vi "PH_USB600x_AnalogReader.set timing mode.vi"(0 "i ref in":refnum<vi>, 1 "Samples per Channel":i32=1000, 2 "Rate":dbl=10000.0 caption="Rate (Hz)" format="%0.2f", 5 "error in (no error)":errorcluster) -> (14 "i ref out":refnum<vi>, 19 "error out":errorcluster)   [LabVIEW 2014, in "PH_USB600x_AnalogReader.lvlib"]
doc: "Sets the timing mode for the scope.\n\nLicense Agreement for this software:\n\nCopyright (C)\nGesellschaft für Schwerionenforschung, GSI\nPlanckstr. 1\n64291 Darmstadt\nGermany\n\nContact: D.Beck@gsi.de \n\nThis program is free software; you can redistribute it and/or modify it under the terms of the GNU General Public License as published by the Free Software Foundation; either version 2 of the license, or (at your option) any later version.\n\nThis program is distributed in the hope that it will be useful, but WITHOUT ANY WARRANTY; without even the implied warranty of MERCHANTABILITY or FITNESS FOR A PARTICULAR PURPOSE. See the GNU General License for more details (http://www.gnu.org).\n\nGesellschaft für Schwerionenforschung, GSI\nPlanckstr. 1, 64291 Darmstadt, Germany\nFor all questions and ideas contact: M.Richter@gsi.de, H.Brand@gsi.de or D.Beck@gsi.de.\nLast update: 17-JUN-2004"
uses:
  PH_USB600x_AnalogReader.lvlib
  PH_Basics/PH_StatusHandler/PH_StatusHandler.Status.ctl
  <vilib>/DAQmx/configure/timing.llb/DAQmx Timing (Sample Clock).vi
  PH_Basics/PH_StatusHandler/PH_StatusHandler.lvlib
  PH_Basics/PH_Common/PH_Common.lvlib
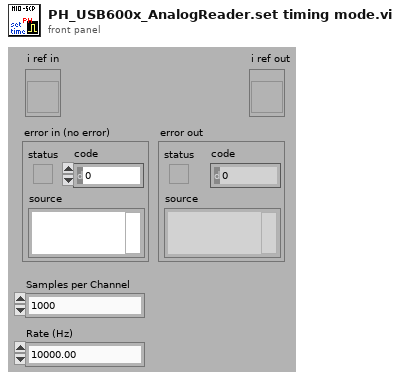
[diagram p1: front panel]
types:
  T1 = typedef "PH_USB600x_AnalogReader.lvlib/PH_USB600x_AnalogReader.i attribute.ctl" = cluster{"GUI Refs":cluster{"Delete":refnum<vi>, "Status":refnum<vi>, "Timeout":refnum<vi>, "Acquire Waveform":refnum<vi>, "Timing":refnum<vi>, "Graph":refnum<vi>, "Prdc Interval":refnum<vi>, "Formula":refnum<vi>}, "Device Settings":cluster{"AIChannel":refnum<k21>, "channelName":string, "Status":T2}, "Timing":T3, "Prdc Interval":dbl, "Lin Scaling":T4, "Data":cluster{"t0":timestamp, dbl}[]}
  T2 = typedef "PH_StatusHandler.lvlib/PH_StatusHandler.Status.ctl" = i16
  T3 = typedef "PH_USB600x_AnalogReader.lvlib/PH_USB600x_AnalogReader.Timing.ctl" = cluster{"Samples per Channel":i32, "Rate":dbl}
  T4 = typedef "PH_USB600x_AnalogReader.lvlib/PH_USB600x_AnalogReader.Lin Scaling.ctl" = cluster{"Slope [Unit/V]":dbl, "Offset [Unit]":dbl, "Y-Unit":string, "Y-Label":string}
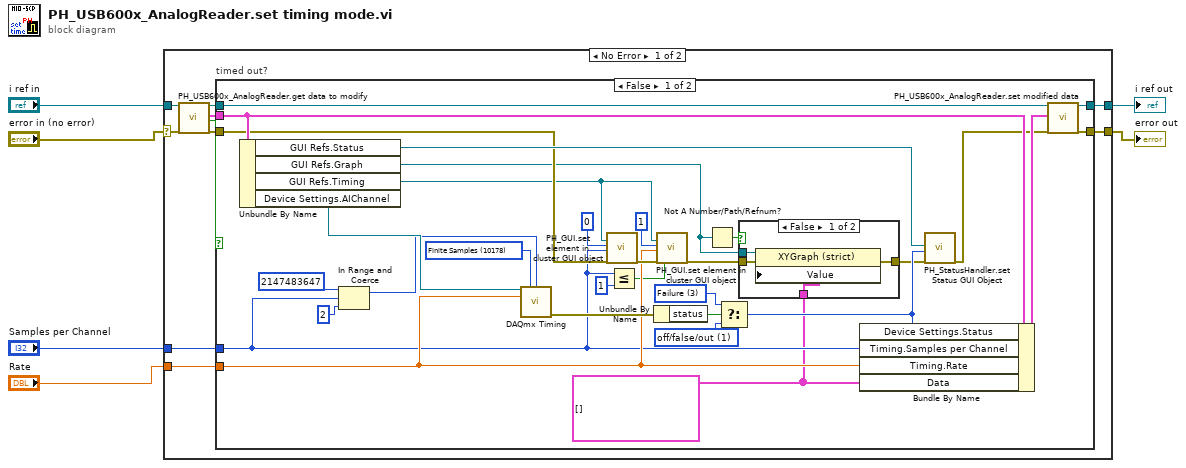
[diagram p0: block diagram]
diagram:
  n1 = case shown="No Error" "error in (no error)" {
    selector: "error in (no error)" -> [w7 w55]
    tunnel: "i ref in" -> [w16 w56]
    tunnel: [w14 w56] -> w5
    tunnel: [w12 w55] -> w4
    tunnel: "Samples per Channel" -> [w9 _]
    tunnel: "Rate" -> [w8 _]
    frame No Error {
      n2 = call "PH_USB600x_AnalogReader.get data to modify.vi"("i ref in"=w16, "error in (no error)"=w7) -> ("i ref out"=w15:refnum<vi>, "i attribute"=w10:T1, "timed out"=w11:bool, "error out"=w13:errorcluster)  [unwired: 14 in]
      n3 = case "timed out?" shown="False" w11 {
        tunnel: [w45 w54] -> w14
        tunnel: w15 -> [w42 w54]
        tunnel: [w41 w53] -> w12
        tunnel: w13 -> [w33 w53]
        tunnel: w10 -> [w44 _]
        tunnel: w9 -> [w23 _]
        tunnel: w8 -> [w31 _]
        frame False {
          w17 = cluster{"t0":timestamp, dbl}[] [] ("Data")
          w38 = T2 1 items=["no info", "off/false/out", "on/true/in", "Failure", "Alarm", "Status 1", "Status 2", "Status 3"] ("Device Settings.Status")
          w39 = T2 3 items=["no info", "off/false/out", "on/true/in", "Failure", "Alarm", "Status 1", "Status 2", "Status 3"] ("Device Settings.Status")
          w46 = 10178 items=["Finite Samples"=10178, "Continuous Samples"=10123, "Hardware Timed Single Point"=12522] ("sample mode")
          n4 = Unbundle By Name(w44) -> ("GUI Refs.Status"=w36:refnum<vi>, "GUI Refs.Graph"=w18:refnum<vi>, "GUI Refs.Timing"=w26:refnum<vi>, "Device Settings.AIChannel"=w43:refnum<k21>)
          n5 = In Range and Coerce(upper limit=2147483647, x=w23, lower limit=2) -> (coerced(x)=w22:i32)  [unwired: 1 out]
          n6 = call-poly <vilib>:"DAQmx Timing.vi"("task/channels in"=w43, "sample mode"=w46, "samples per channel"=w22, "rate"=w31) -> ("error out"=w37:errorcluster)  [unwired: 10 in, 1 out]
          n7 = call "PH_GUI.set element in cluster GUI object.vi"("Cluster Ref"=w26, "Cluster index"=0, "Value"=w23, "error in (no error)"=w33) -> ("error out"=w32:errorcluster)  [unwired: 15 in]
          n8 = Less Or Equal?(x=w23, y=1) -> (x <= y?=w29:bool)
          n9 = Unbundle By Name(w37) -> ("status"=w40:bool)
          n10 = call "PH_GUI.set element in cluster GUI object.vi"("Cluster Ref"=w26, "Cluster index"=1, "Value"=w31, "error in (no error)"=w32, "Grayed out? (false)"=w29) -> ("error out"=w21:errorcluster)  [unwired: 14 in]
          n11 = Not A Number/Path/Refnum?(number/path/refnum=w18) -> (NaN/Path/Refnum?=w19:bool)
          n12 = Select(t=w39, s=w40, f=w38) -> (s? t:f=w34:T2)
          n13 = case shown="False" w19 {
            tunnel: w21 -> [w51 w52]
            tunnel: [w50 w52] -> w20
            tunnel: w18 -> [w49 _]
            tunnel: w17 -> [w48 _]
            frame False {
              n14 = property class="XYGraph (strict)"(reference=w49, error in=w51, "Value"=w48) -> (error out=w50:errorcluster)  [unwired: 1 out]
            }
            frame True {
            }
          }
          n15 = Bundle By Name(cluster=w44, "Device Settings.Status"=w34, "Timing.Samples per Channel"=w23, "Timing.Rate"=w31, "Data"=w17) -> (w47:T1)
          n16 = call "PH_StatusHandler.set Status GUI Object.vi"("PH Status Ref"=w36, "Value"=w34, "error in (no error)"=w20) -> ("error out"=w35:errorcluster)  [unwired: 16 in]
          n17 = call "PH_USB600x_AnalogReader.set modified data.vi"("i ref in"=w42, "i attribute"=w47, "error in (no error)"=w35) -> ("i ref out"=w45:refnum<vi>, "error out"=w41:errorcluster)  [unwired: 15 in]
        }
        frame True {
        }
      }
    }
    frame Error {
    }
  }
  "error out" <- w4
  "i ref out" <- w5
